vi "InteractiveDrawArmPath.vi"(6 "PathPercent":dbl(slide) scale=0.0..1.0, 7 "RobotDimensions":T2, 8 "AvoidancePolygon":cluster{"X":dbl[], "Y":dbl[]}, 9 "MaxRadiusCircle":cluster{"X":dbl[], "Y":dbl[]}, 10 "MinRadiusCircle":cluster{"X":dbl[], "Y":dbl[]}, 11 "Path":T3[](array[typedef])) -> (0 "RawArmPosition":T1, 1 "Arm Position":cluster{"X":dbl[], "Y":dbl[]}[](graph)=[{"X"=[-15.5, -15.5, -6.0, -6.0, 6.0, 6.0, 15.5, 15.5, 45.5, 45.5, 6.0, 6.0, -6.0, -6.0, -45.5, -45.5, -15.5], "Y"=[0.0, 7.0, 7.0, 12.0, 12.0, 7.0, 7.0, 0.0, 0.0, 90.0, 90.0, 24.0, 24.0, 90.0, 90.0, 0.0, 0.0]}, {"X"=array[361 elements], "Y"=array[361 elements]}, {"X"=array[361 elements], "Y"=array[361 elements]}, {"X"=[0.0, 21.000000000000004], "Y"=[44.25, 15.0]}, {"X"=[21.000000000000004, 26.99999809759101], "Y"=[15.0, 14.995222039735602]}, {"X"=[22.499999524397754, 22.499999524397758, 19.500000475602256, 19.500000475602253], "Y"=[14.9988055099339, 2.9988055099339004, 3.0011944900660996, 15.0011944900661]}])   [LabVIEW 2018]
uses:
  TypeDefs/ArmCoordinate.ctl
  TypeDefs/ConfigComponents/Config_Dimensions.ctl
  TypeDefs/ArmAbsolutePosition.ctl
panel:
  in  "Wrist Length (in)":dbl=6.0
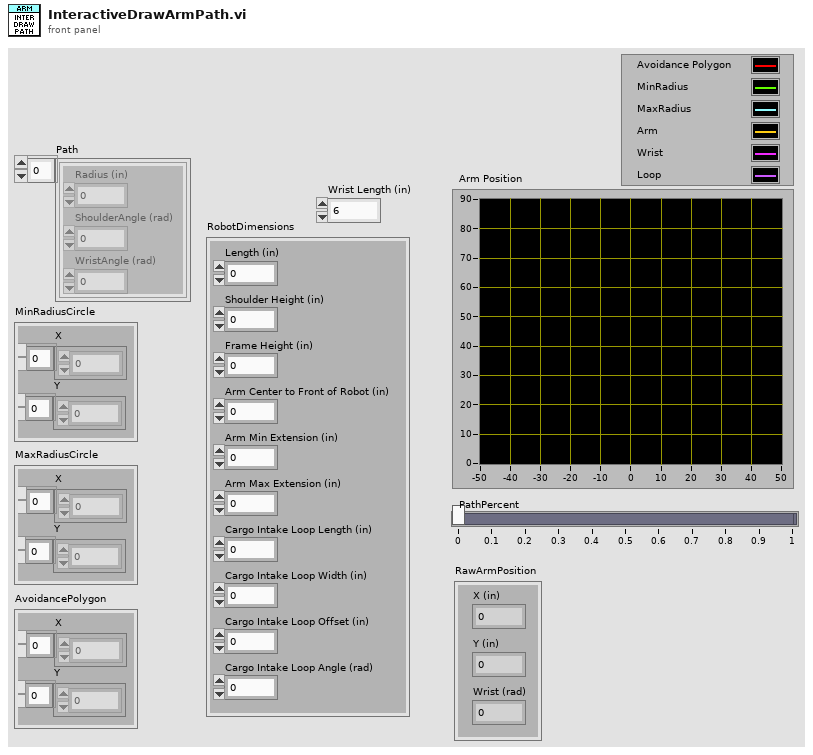
[diagram p1: front panel]
types:
  T1 = typedef "ArmAbsolutePosition.ctl" = cluster{"X (in)":dbl, "Y (in)":dbl, "Wrist (rad)":dbl}
  T2 = typedef "Config_Dimensions.ctl" = cluster{"Length (in)":dbl, "Shoulder Height (in)":dbl, "Frame Height (in)":dbl, "Arm Center to Front of Robot (in)":dbl, "Arm Min Extension (in)":dbl, "Arm Max Extension (in)":dbl, "Cargo Intake Loop Length (in)":dbl, "Cargo Intake Loop Width (in)":dbl, "Cargo Intake Loop Offset (in)":dbl, "Cargo Intake Loop Angle (rad)":dbl}
  T3 = typedef "ArmCoordinate.ctl" = cluster{"Radius (in)":dbl, "ShoulderAngle (rad)":dbl, "WristAngle (rad)":dbl}
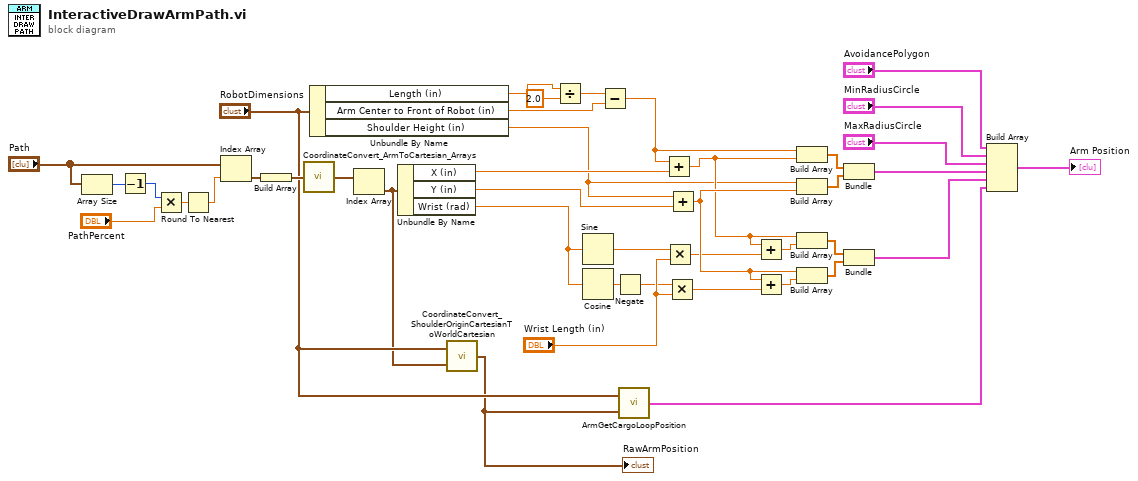
[diagram p0: block diagram]
diagram:
  n1 = Array Size(array="Path") -> (size(s)=w42:i32)
  n2 = Decrement(x=w42) -> (x-1=w40:i32)
  n3 = Multiply(x=w40, y="PathPercent") -> (x*y=w39:dbl)
  n4 = Round To Nearest(number=w39) -> (nearest integer value=w38:dbl)
  n5 = Index Array(array="Path", index=w38) -> (element=w36:T3)
  n6 = Build Array(w36) -> (w35:T3[])
  n7 = call "CoordinateConvert_ArmToCartesian_Arrays.vi"("ArmCoordinates"=w35) -> ("XYPoints"=w18:T1[])
  n8 = Unbundle By Name("RobotDimensions") -> ("Length (in)"=w8:dbl, "Arm Center to Front of Robot (in)"=w5:dbl, "Shoulder Height (in)"=w6:dbl)
  n9 = Index Array(array=w18) -> (element=w2:T1)  [unwired: 1 in]
  n10 = Unbundle By Name(w2) -> ("X (in)"=w34:dbl, "Y (in)"=w33:dbl, "Wrist (rad)"=w30:dbl)
  n11 = call "CoordinateConvert_ShoulderOriginCartesianToWorldCartesian.vi"("ArmPositionRelativeToShoulderIn"=w2, "RobotDimensions"="RobotDimensions") -> ("ArmPosition"=w1:T1)
  "RawArmPosition" <- w1
  n12 = Divide(x=w8, y=2.0) -> (x/y=w9:dbl)
  n13 = Sine(x=w30) -> (sin(x)=w29:dbl)
  n14 = Cosine(x=w30) -> (cos(x)=w28:dbl)
  n15 = Subtract(x=w9, y=w5) -> (x-y=w7:dbl)
  n16 = Negate(x=w28) -> (-x=w11:dbl)
  n17 = call "ArmGetCargoLoopPosition.vi"("ArmAbsolutePose"=w1, "RobotDimensions"="RobotDimensions") -> ("CargoLoopPoints"=w4:cluster{dbl[], dbl[]})
  n18 = Add(x=w7, y=w34) -> (x+y=w14:dbl)
  n19 = Multiply(x=w29, y="Wrist Length (in)") -> (x*y=w13:dbl)
  n20 = Multiply(x=w11, y="Wrist Length (in)") -> (x*y=w17:dbl)
  n21 = Add(x=w6, y=w33) -> (x+y=w16:dbl)
  n22 = Add(x=w14, y=w13) -> (x+y=w12:dbl)
  n23 = Add(x=w16, y=w17) -> (x+y=w15:dbl)
  n24 = Build Array(w7, w14) -> (w32:dbl[])
  n25 = Build Array(w6, w16) -> (w31:dbl[])
  n26 = Build Array(w14, w12) -> (w26:dbl[])
  n27 = Build Array(w16, w15) -> (w25:dbl[])
  n28 = Bundle(w32, w31) -> (w21:cluster{dbl[], dbl[]})  [unwired: 1 in]
  n29 = Bundle(w26, w25) -> (w20:cluster{dbl[], dbl[]})  [unwired: 1 in]
  n30 = Build Array("AvoidancePolygon", "MinRadiusCircle", "MaxRadiusCircle", w21, w20, w4) -> (→"Arm Position":cluster{"X":dbl[], "Y":dbl[]}[])
